vi "Read Column Headers.vi"(11 "Base Display Configuration in":refnum<class "Base Display Configuration.lvclass">) -> (2 "Column Headers":string[](array[string]))   [LabVIEW 2016, in "Assert API Components.lvlib" / "Assert Display.lvlib" / "Main Display.lvlib" / "Base Display Configuration.lvclass"]
uses:
  Base Display Configuration.lvclass
  Base Display Configuration.lvclass/Base Display Configuration.ctl
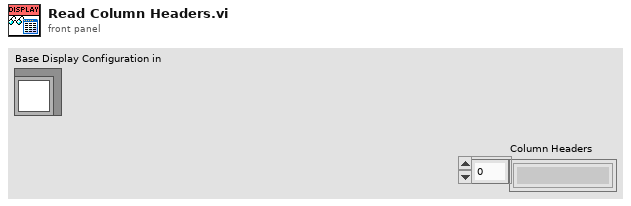
[diagram p1: front panel]
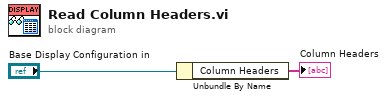
[diagram p0: block diagram]
diagram:
  n1 = Unbundle By Name("Base Display Configuration in") -> ("Column Headers"=→"Column Headers":string[])
